vi "Router - CVT FGV.vi"(7 "FGV Command":enum16{"Init", "Write Table", "Read Table"}(ring), 8 "error in (no error)":errorcluster, 9 "Tag Array Write":dbl[](array[numeric]), 10 "Tag Name":string, 11 "CVT Tags to Create":T1={"Tags"=[{"Data Type"=enum."Array of Double", "Name"="Slave 1", "Value"="", "Description"=""}, {"Data Type"=enum."Array of Double", "Name"="Slave 2", "Value"="", "Description"=""}], "Group Listings"=[]}) -> (0 "error out":errorcluster, 1 "Tag Array Read":dbl[](array[numeric]))   [LabVIEW 2016]
uses:
  <vilib>/NI/Current Value Table/Type Defs/File Format.ctl
  <vilib>/NI/Current Value Table/Type Defs/Single Tag.ctl
  <vilib>/NI/Current Value Table/Type Defs/Data Types.ctl
  <vilib>/NI/Current Value Table/Type Defs/Tag Grouping set.ctl
  <vilib>/NI/Current Value Table/DataTypes/Array of Double_Write.vi
  <vilib>/NI/Current Value Table/DataTypes/Array of Double_Read.vi
  <vilib>/NI/Current Value Table/Type to Enum.vi
  <vilib>/NI/Current Value Table/DataTypes/Array of Double_Type To Enum.vi
  <vilib>/NI/Current Value Table/FGVs/CVT Globals.vi
  <vilib>/NI/Current Value Table/FGVs/Tag Memory.vi
  <vilib>/NI/Current Value Table/Memory Block.vi
  <vilib>/NI/Current Value Table/DataTypes/Array of Double_Memory Block.vi
  <vilib>/NI/Current Value Table/Current Value Table.lvlib
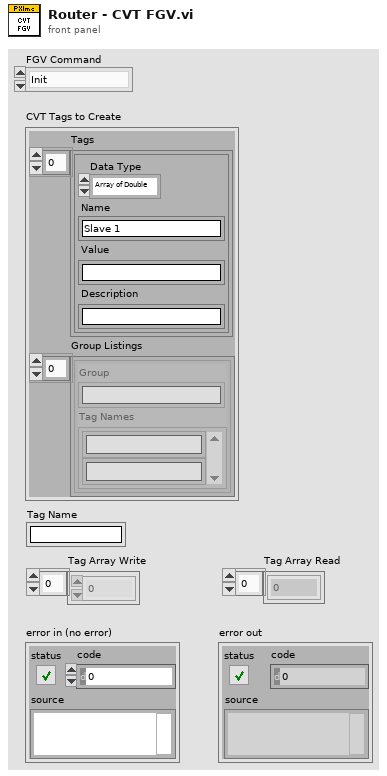
[diagram p1: front panel]
types:
  T1 = typedef "Current Value Table.lvlib/File Format.ctl" = cluster{"Tags":T2[], "Group Listings":T4[]}
  T2 = typedef "Current Value Table.lvlib/Single Tag.ctl" = cluster{"Data Type":T3, "Name":string, "Value":string, "Description":string}
  T3 = typedef "Current Value Table.lvlib/Data Types.ctl" = enum16{"Double", "Single", "I64", "I32", "I16", "I8", "U64", "U32", "U16", "U8", "String", "Boolean", "Array of U8", "Array of U16", "Array of U32", "Array of U64", "Array of I64", "Array of I32", "Array of I16", "Array of I8", "Array of Double", "Array of Single", "Array of Boolean", "Array of String"}
  T4 = typedef "Current Value Table.lvlib/Tag Grouping set.ctl" = cluster{"Group":string, "Tag Names":string[]}
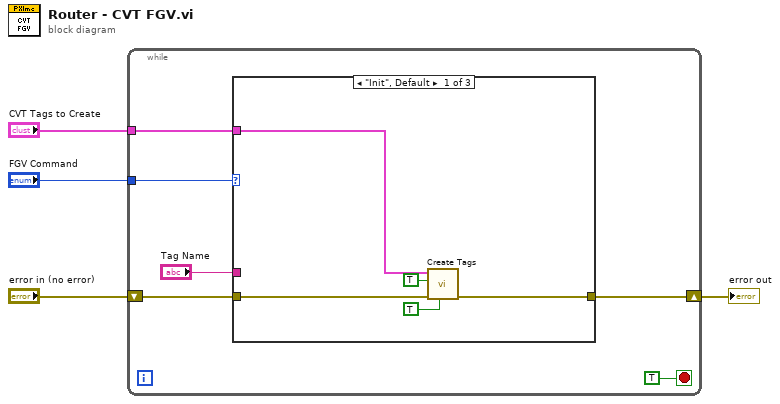
[diagram p0: block diagram]
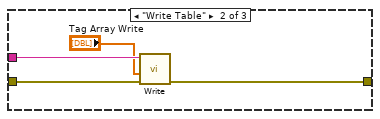
[diagram p2: hidden frame]
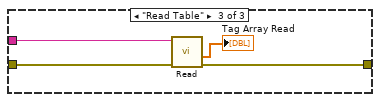
[diagram p3: hidden frame]
diagram:
  n1 = while {
    tunnel: "FGV Command" -> [w9]
    shift-right: [w8] -> w2
    shift-left: "error in (no error)" -> [w7]
    tunnel: "CVT Tags to Create" -> [w5]
    stop <- TRUE stop-if-true
    n2 = case shown="\"Init\", Default" w9 {
      tunnel: [w14 w18 w21] -> w8
      tunnel: w7 -> [w13 w19 w22]
      tunnel: "Tag Name" -> [_ w17 w23]
      tunnel: w5 -> [w12 _ _]
      frame "Init", Default {
        n3 = call <vilib>:"Create Tags.vi"("Overwrite Duplicates? (F)"=TRUE, "error in (no error)"=w13, "Clear Table? (F)"=TRUE, "CVT Tags to Create"=w12) -> ("error out"=w14:errorcluster)  [unwired: 7 in]
      }
      frame "Write Table" {
        n4 = call-poly <vilib>:"Write.vi"("error in (no error)"=w19, "Value"="Tag Array Write", "Tag Name"=w17) -> ("error out"=w18:errorcluster)  [unwired: 8 in]
      }
      frame "Read Table" {
        n5 = call-poly <vilib>:"Read.vi"("error in (no error)"=w22, "Tag Name"=w23) -> ("error out"=w21:errorcluster, "Value"=→"Tag Array Read":dbl[])  [unwired: 8 in]
      }
    }
  }
  "error out" <- w2
